vi "evalLoopTimeOutOfRangeLimit.vi"(8 "error in (no error)":errorcluster, 11 "LoopTimer in":refnum<class "LoopTimer.lvclass">) -> (0 "error out":errorcluster, 3 "LoopTimer out":refnum<class "LoopTimer.lvclass">)   [LabVIEW 2013, in "ComponentData.lvlib" / "LoopTimer.lvclass"]
uses:
  <userlib>/Common/Component/common_application/RT/ComponentData/LoopTimer/LoopTimer.lvclass
  <userlib>/Common/Component/common_application/RT/ComponentData/LoopTimer/LoopTimer.lvclass/LoopTimer.ctl
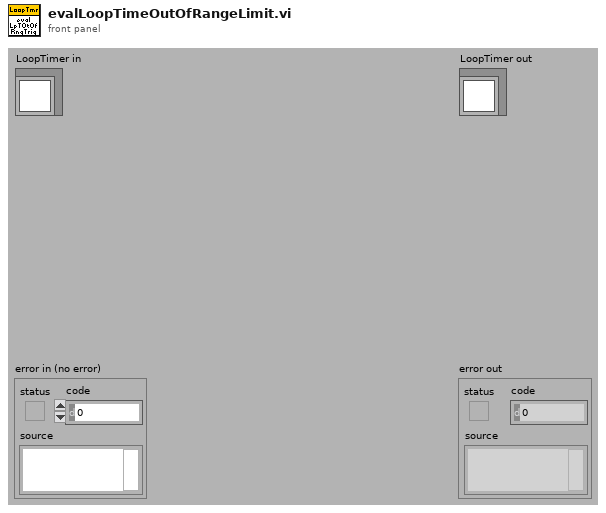
[diagram p1: front panel]
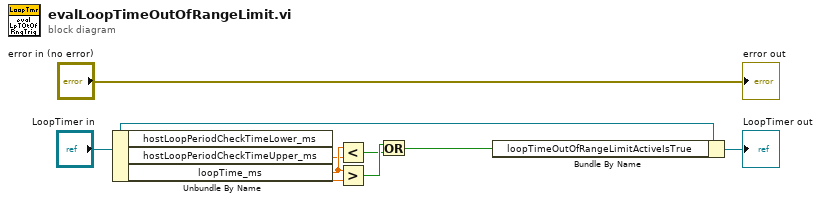
[diagram p0: block diagram]
diagram:
  n1 = Unbundle By Name("LoopTimer in") -> ("hostLoopPeriodCheckTimeLower_ms"=w4:dbl, "hostLoopPeriodCheckTimeUpper_ms"=w5:dbl, "loopTime_ms"=w6:dbl)
  n2 = Less?(x=w6, y=w4) -> (x < y?=w2:bool)
  n3 = Greater?(x=w6, y=w5) -> (0:w3:bool)
  n4 = Or(x=w3, y=w2) -> (x .or. y?=w1:bool)
  n5 = Bundle By Name(cluster="LoopTimer in", "loopTimeOutOfRangeLimitActiveIsTrue"=w1) -> (→"LoopTimer out":refnum<class "LoopTimer.lvclass">)
  "error out" <- "error in (no error)"
